vi "Read Condition.vi"(11 "Interlock Bool in":refnum<class "Interlock Bool.lvclass">) -> (2 "Interlock Condition":bool, 3 "Interlock Bool out":refnum<class "Interlock Bool.lvclass">)   [LabVIEW 2015, in "Interlocks.lvlib" / "Interlock Bool.lvclass"]
uses:
  Interlock Bool.lvclass
  Interlock Bool.lvclass/Interlock Bool.ctl
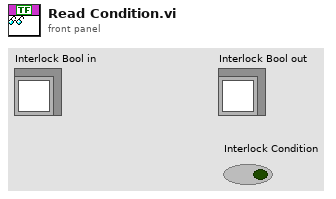
[diagram p1: front panel]
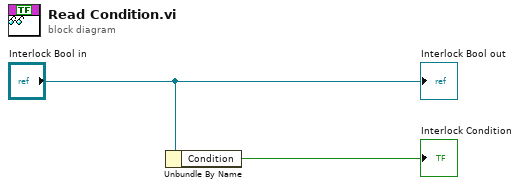
[diagram p0: block diagram]
diagram:
  n1 = Unbundle By Name("Interlock Bool in") -> ("Condition"=→"Interlock Condition":bool)
  "Interlock Bool out" <- "Interlock Bool in"
